vi "Power Output Flatten Test Parameters.vi"(7 "Test Configuration (\"\")":string, 9 "error in (no error)":errorcluster, 10 "Parameter Variant":variant) -> (1 "error out":errorcluster, 2 "Parameter String":string)   [LabVIEW 2011]
uses:
  Power Output Version.vi
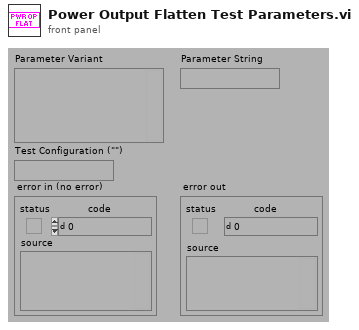
[diagram p1: front panel]
types:
  T1 = typedef "Power Output Test Parameters.ctl" = cluster{"Stimulus":T2, "Measurement":T3, "Display":T7, "Limit":T8, "Calibration":T9}
  T2 = typedef "Power Output Stimulus Parameters.ctl" = cluster{"Frequency Type":enum16{"Band Edges", "Custom"}, "Frequency Ranges":cluster{"Start (MHz)":dbl, "Stop (MHz)":dbl}[], "TX 1 Frequency (MHz)":cluster{"Min":dbl, "Max":dbl}, "TX 2 Frequency (MHz)":cluster{"Min":dbl, "Max":dbl}, "RX Frequency (MHz)":cluster{"Min":dbl, "Max":dbl}, "Pad Model Number":string, "Pad Serial Number":string, "Pad Values":dbl[][][]}
  T3 = typedef "Power Output Measurement Parameters.ctl" = cluster{"DUT Port":T4, "Direction":T5, "Frequency Step Size":T6}
  T4 = typedef "DUTport.ctl" = enum16{"Port 1", "Port 2"}
  T5 = typedef "MeasMode.ctl" = u16
  T6 = typedef "PIM Sweep Step Size.ctl" = u16
  T7 = typedef "Power Output Display Parameters.ctl" = cluster{"Frequency":cluster{"Min":dbl, "Max":dbl}, "Power":cluster{"Min":i32, "Max":i32}}
  T8 = typedef "Power Output Limit Parameters.ctl" = cluster{"Min Power (dBm)":dbl}
  T9 = typedef "Power Output Calibration State.ctl" = cluster{"Calibrated?":bool}
  T10 = typedef "OGAB Version.ctl" = cluster{"Version":string, "Build Number":u32, "Build Date/Time":dbl}
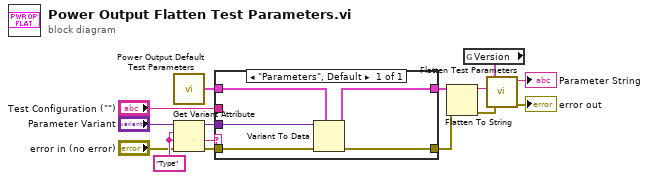
[diagram p0: block diagram]
diagram:
  w14 = "Type" ("name")
  n1 = call "Power Output Default Test Parameters.vi"() -> ("Default Power Output Test Parameters"=w1:T1)
  n2 = Get Variant Attribute(Variant="Parameter Variant", name=w14, default value (empty Variant)=w14, error in="error in (no error)") -> (duplicate Variant=w5:variant, value=w4:string, error out=w6:errorcluster)  [unwired: 1 out]
  n3 = case shown="\"Parameters\", Default" w4 {
    tunnel: w5 -> [w20]
    tunnel: w1 -> [w16]
    tunnel: [w17] -> w2
    tunnel: [w19] -> w3
    tunnel: w6 -> [w18]
    tunnel: "Test Configuration (\"\")" -> [_]
    frame "Parameters", Default {
      n4 = Variant To Data(error in=w18, type=w16, Variant=w20) -> (data=w17:T1, error out=w19:errorcluster)
    }
  }
  n5 = Flatten To String(anything=w2, error in (no error)=w3) -> (data string=w13:string, error out=w11:errorcluster)  [unwired: 3 out]
  n6 = global read "Power Output Version.vi" "Version"() -> (w12:T10)
  n7 = call "Flatten Test Parameters.vi"("error in (no error)"=w11, "Flattened Test Parameters (\"\")"=w13, "Test Version"=w12) -> ("error out"=→"error out":errorcluster, "Flattened Test Parameters with Version"=→"Parameter String":string)  [unwired: 3 out]
